vi "TranslateVoltages.vi"(0 "Input arm settings":T2(array[cluster]), 1 "Input channel":T3, 2 "Reading / V":dbl, 3 "error in (no error)":errorcluster) -> (4 "Output / V":dbl=nan, 5 "Output / C":dbl=nan, 7 "Output is temperature?":bool, 8 "Output":dbl=nan, 9 "error out":errorcluster)   [LabVIEW 2015]
doc: "Use the constants defined in the data cluster to translate a voltage into a temperature if required"
uses:
  Driver/Typedefs/InputChannelTypedef.ctl
  controls/ChannelSettings.ctl
  Driver/YbTempCtrl.lvlib
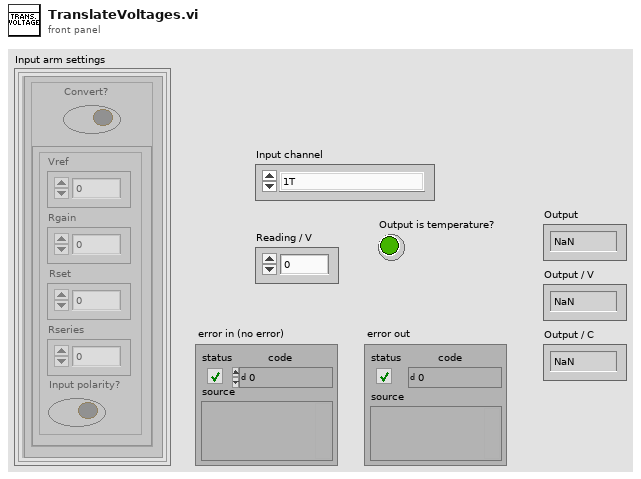
[diagram p1: front panel]
types:
  T1 = typedef "ChannelSettings.ctl" = cluster{"Convert?":bool, "Config":cluster{"Vref":dbl, "Rgain":dbl, "Rset":dbl, "Rseries":dbl, "Input polarity?":bool}}
  T2 = cluster{"Enum string":string, "Enum ID":i16, "Input arm settings":T1}[]
  T3 = typedef "YbTempCtrl.lvlib/InputChannelTypedef.ctl" = enum16{"1T", "2T", "TMP", "POW"}
  T4 = cluster{"Enum string":string, "Enum ID":i16, "Input arm settings":T1}
  T5 = cluster{"Vref":dbl, "Rgain":dbl, "Rset":dbl, "Rseries":dbl, "Input polarity?":bool}
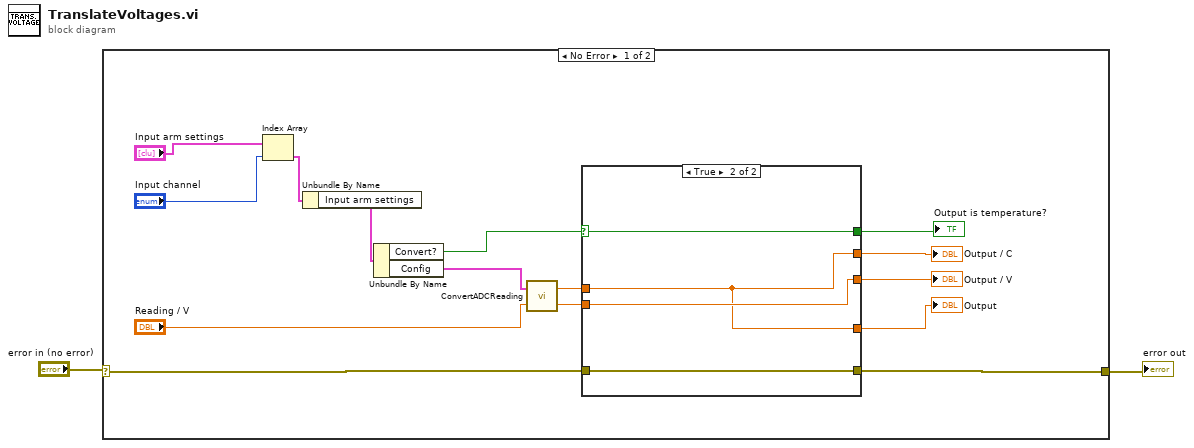
[diagram p0: block diagram]
diagram:
  n1 = case shown="No Error" "error in (no error)" {
    selector: "error in (no error)" -> [w14 w26]
    tunnel: [w15 w26] -> w1
    frame No Error {
      n2 = Index Array(array="Input arm settings", index="Input channel") -> (element=w11:T4)
      n3 = Unbundle By Name(w11) -> ("Input arm settings"=w10:T1)
      n4 = Unbundle By Name(w10) -> ("Convert?"=w17:bool, "Config"=w9:T5)
      n5 = call "ConvertADCReading.vi"("Reading / V"="Reading / V", "Input arm settings"=w9) -> ("Voltage / V"=w6:dbl, "Temperature / C"=w7:dbl)
      n6 = case shown="True" w17 {
        selector: w17 -> [w21 w25]
        tunnel: [w21 w25] -> w16
        tunnel: [w20 w24] -> w15
        tunnel: w14 -> [w20 w24]
        tunnel: w7 -> [w19 w22]
        tunnel: w6 -> [w18 w23]
        tunnel: [w19 w22] -> w5
        tunnel: [w18 w23] -> w4
        tunnel: [w18 w22] -> w3
        frame False {
        }
        frame True {
        }
      }
      "Output is temperature?" <- w16
      "Output" <- w3
      "Output / V" <- w4
      "Output / C" <- w5
    }
    frame Error {
    }
  }
  "error out" <- w1
